vi "ZyklussteuerungGV-05-17.vi"(0 "Traps/MachKoeff0":dbl[](array[numeric]), 1 "DIOsNummern":cluster{"DIOsMod2BNr":i32[]}[](array[cluster]), 2 "error in":errorcluster, 5 "Traps/MachKoeff1":dbl[](array[numeric]), 9 "Traps/MachKoeff2":dbl[](array[numeric]), 11 "Schieberegister":T1, 12 "Zeitpunkte/Setpoints":T3 {"FPGAPID"."proportional gain (Kc)" format="%.11g"; "FPGAPID"."integral gain (Kc*Ts/Ti)" format="%.11g"; "FPGAPID"."derivative gain (Kc*Td/Ts)" format="%.11g"}, 13 "FPGA VI Reference In":refnum<k20>, 14 "MachKoeffs":T2) -> (4 "Schieberegister":T1, 8 "error out":errorcluster)   [LabVIEW 2010]
uses:
  <vilib>/rvi/errors/niLvFpgaWhatHappensToTopLevelVI.ctl
  <vilib>/rvi/interface/common/niFpgaNodeNameForErrorReporting.ctl
  <vilib>/rvi/errors/niLvFpgaAdjustHostInterfaceError.vi
  <vilib>/rvi/interface/nirviReadWriteControl/nirviReadWriteControl.xnode
  GVZwangs.vi
  GVHorstSP.vi
  GVHeizenLH.vi
  GVVentilposition.vi
  GVZeitenZyklen.vi
  GVZwangsMPV.vi
  GVZwangsMPVPos.vi
  C:/Users/HAGAR-IV/Desktop/Zeugs/Johnny/pertrasgc fpga/FPGA-Programm-05-17.vi
  <vilib>/RVI Host/nirviSupport.llb/nirviErrorClusterFromErrorCode.vi
  C:/Users/HAGAR-IV/Desktop/Zeugs/markus/version feb 2012/FPGA Bitfiles/pertrasgcfpga2_FPGATarget_FPGA-Programm-05_A75D3647.lvbitx
  NiFpgaLv.dll
  <vilib>/Utility/error.llb/Error Cluster From Error Code.vi
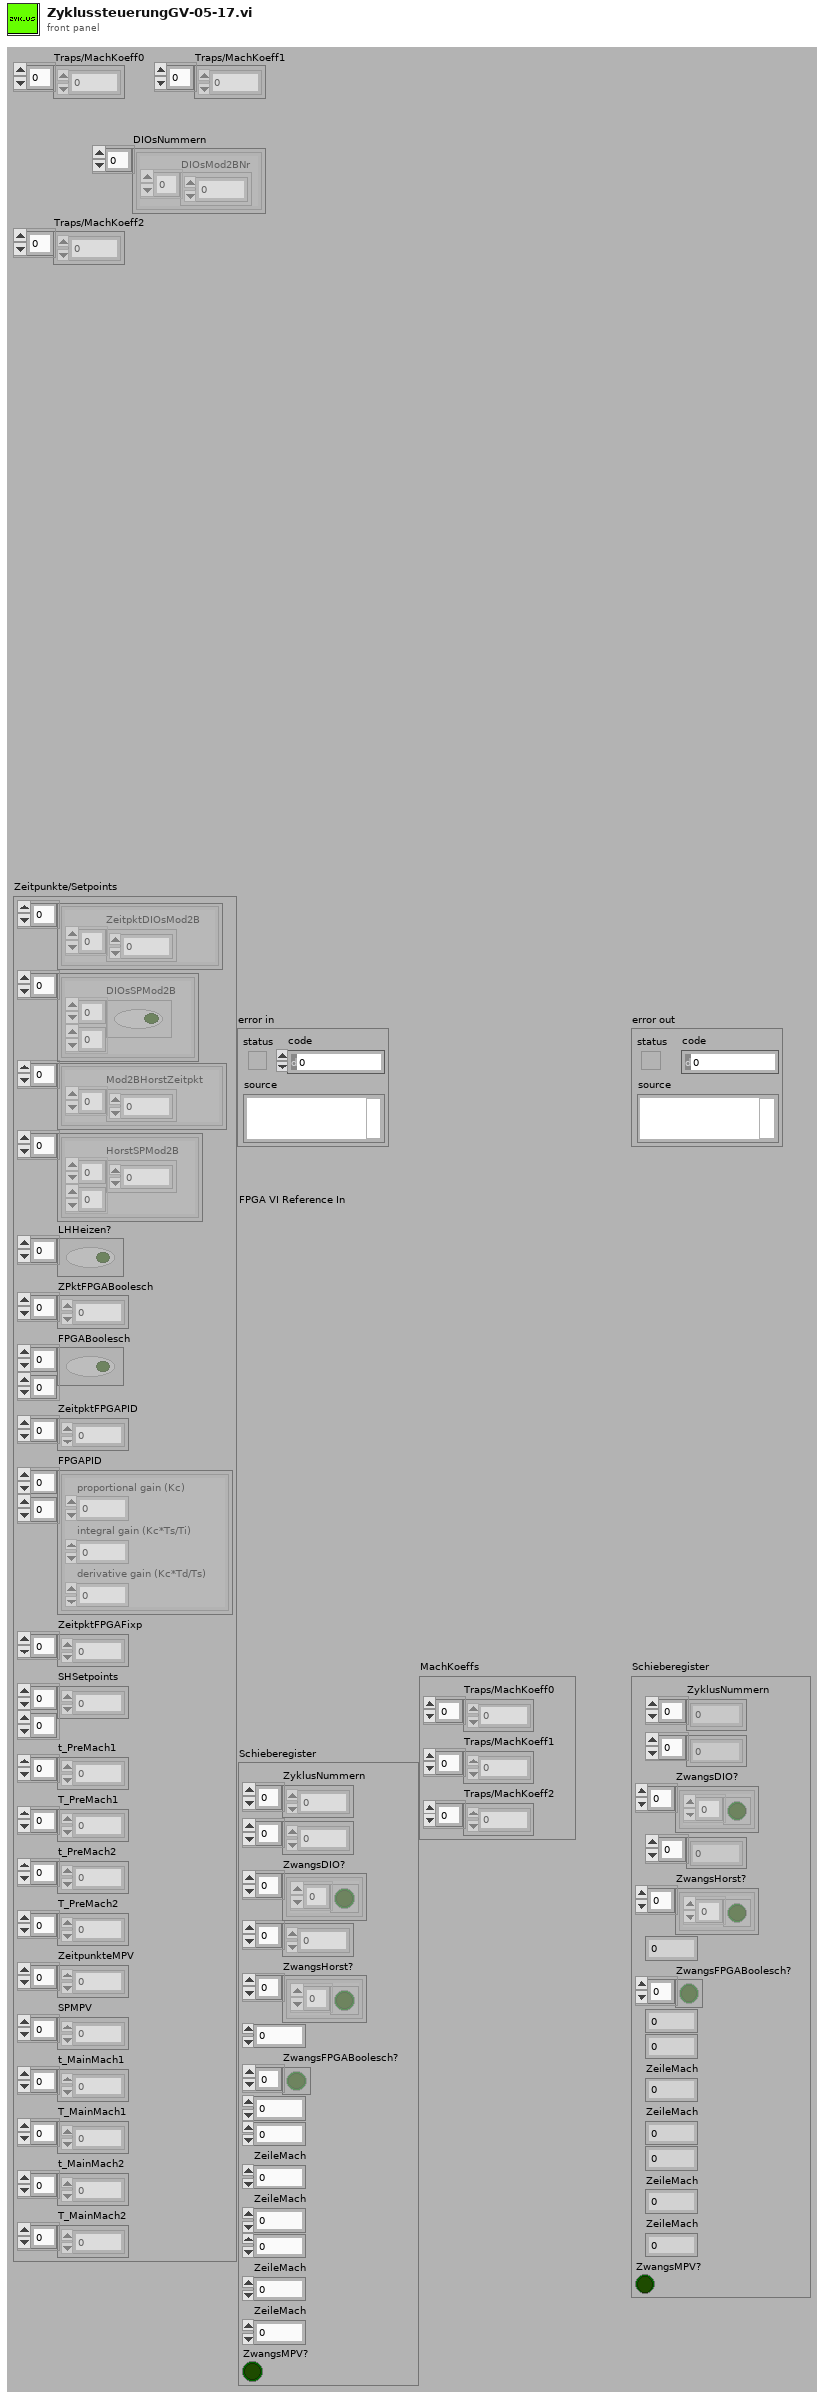
[diagram p1: front panel]
types:
  T1 = cluster{"ZyklusNummern":i32[], i32[], "ZwangsDIO?":cluster{bool[]}[], i32[], "ZwangsHorst?":cluster{bool[]}[], i32, "ZwangsFPGABoolesch?":bool[], i32, i32, "ZeileMach":i32, "ZeileMach":i32, i32, "ZeileMach":i32, "ZeileMach":i32, "ZwangsMPV?":bool}
  T2 = cluster{"Traps/MachKoeff0":dbl[], "Traps/MachKoeff1":dbl[], "Traps/MachKoeff2":dbl[]}
  T3 = cluster{cluster{"ZeitpktDIOsMod2B":dbl[]}[], cluster{"DIOsSPMod2B":bool[][]}[], cluster{"Mod2BHorstZeitpkt":dbl[]}[], cluster{"HorstSPMod2B":dbl[][]}[], "LHHeizen?":bool[], "ZPktFPGABoolesch":dbl[], "FPGABoolesch":bool[][], "ZeitpktFPGAPID":dbl[], "FPGAPID":cluster{"proportional gain (Kc)":fxp<+/-,16,8>, "integral gain (Kc*Ts/Ti)":fxp<+/-,16,8>, "derivative gain (Kc*Td/Ts)":fxp<+/-,16,8>}[][], "ZeitpktFPGAFixp":dbl[], "SHSetpoints":dbl[][], "t_PreMach1":dbl[], "T_PreMach1":dbl[], "t_PreMach2":dbl[], "T_PreMach2":dbl[], "ZeitpunkteMPV":dbl[], "SPMPV":i32[], "t_MainMach1":dbl[], "T_MainMach1":dbl[], "t_MainMach2":dbl[], "T_MainMach2":dbl[]}
  T4 = cluster{"proportional gain (Kc)":fxp<+/-,16,8>, "integral gain (Kc*Ts/Ti)":fxp<+/-,16,8>, "derivative gain (Kc*Td/Ts)":fxp<+/-,16,8>}[][]
  T5 = typedef "niFpgaNodeNameForErrorReporting.ctl" = enum16{"Open FPGA VI Reference", "Read/Write Control", "Invoke Method: Abort", "Invoke Method: Acknowledge IRQ", "Invoke Method: Download", "Invoke Method: FIFO.Configure", "Invoke Method: FIFO.Read", "Invoke Method: FIFO.Start", "Invoke Method: FIFO.Stop", "Invoke Method: FIFO.Write", "Invoke Method: Reset", "Invoke Method: Run", "Invoke Method: Wait on IRQ", "Close FPGA VI Reference"}
  T6 = typedef "niLvFpgaWhatHappensToTopLevelVI.ctl" = enum16{"top level VI scripted behind XNode", "top level VI inlined behind XNode"}
  T7 = cluster{"[0]":bool, "[1]":bool, "[2]":bool, "[3]":bool, "[4]":bool, "[5]":bool, "[6]":bool, "[7]":bool, "[8]":bool, "[9]":bool, "[10]":bool, "[11]":bool, "[12]":bool, "[13]":bool, "[14]":bool, "[15]":bool, "[16]":bool, "[17]":bool, "[18]":bool, "[19]":bool, "[20]":bool, "[21]":bool, "[22]":bool, "[23]":bool, "[24]":bool, "[25]":bool, "[26]":bool, "[27]":bool, "[28]":bool, "[29]":bool, "[30]":bool, "[31]":bool}
  T8 = cluster{"[0]":bool, "[1]":bool, "[2]":bool, "[3]":bool, "[4]":bool, "[5]":bool}
  T9 = cluster{"proportional gain (Kc)":fxp<+/-,16,8>, "integral gain (Kc*Ts/Ti)":fxp<+/-,16,8>, "derivative gain (Kc*Td/Ts)":fxp<+/-,16,8>}[]
  T10 = cluster{"FPGAPID[0]":cluster{"proportional gain (Kc)":fxp<+/-,16,8>, "integral gain (Kc*Ts/Ti)":fxp<+/-,16,8>, "derivative gain (Kc*Td/Ts)":fxp<+/-,16,8>}, "FPGAPID[1]":cluster{"proportional gain (Kc)":fxp<+/-,16,8>, "integral gain (Kc*Ts/Ti)":fxp<+/-,16,8>, "derivative gain (Kc*Td/Ts)":fxp<+/-,16,8>}, "FPGAPID[2]":cluster{"proportional gain (Kc)":fxp<+/-,16,8>, "integral gain (Kc*Ts/Ti)":fxp<+/-,16,8>, "derivative gain (Kc*Td/Ts)":fxp<+/-,16,8>}, "FPGAPID[3]":cluster{"proportional gain (Kc)":fxp<+/-,16,8>, "integral gain (Kc*Ts/Ti)":fxp<+/-,16,8>, "derivative gain (Kc*Td/Ts)":fxp<+/-,16,8>}, "FPGAPID[4]":cluster{"proportional gain (Kc)":fxp<+/-,16,8>, "integral gain (Kc*Ts/Ti)":fxp<+/-,16,8>, "derivative gain (Kc*Td/Ts)":fxp<+/-,16,8>}, "FPGAPID[5]":cluster{"proportional gain (Kc)":fxp<+/-,16,8>, "integral gain (Kc*Ts/Ti)":fxp<+/-,16,8>, "derivative gain (Kc*Td/Ts)":fxp<+/-,16,8>}}
  T11 = cluster{"proportional gain (Kc)":fxp<+/-,16,8>, "integral gain (Kc*Ts/Ti)":fxp<+/-,16,8>, "derivative gain (Kc*Td/Ts)":fxp<+/-,16,8>}
  T12 = cluster{"USetp [V]Mach1":fxp<+/-,16,6>, "[1]":fxp<+/-,16,4>, "[2]":fxp<+/-,16,4>, "[3]":fxp<+/-,16,4>, "[4]":fxp<+/-,16,4>, "[5]":fxp<+/-,16,4>, "[6]":fxp<+/-,16,4>, "[7]":fxp<+/-,16,4>, "[8]":fxp<+/-,16,4>}
  T13 = cluster{"SpannungenSH[V][0]":fxp<+/-,16,4>, "SpannungenSH[V][1]":fxp<+/-,16,4>, "SpannungenSH[V][2]":fxp<+/-,16,4>, "SpannungenSH[V][3]":fxp<+/-,16,4>}
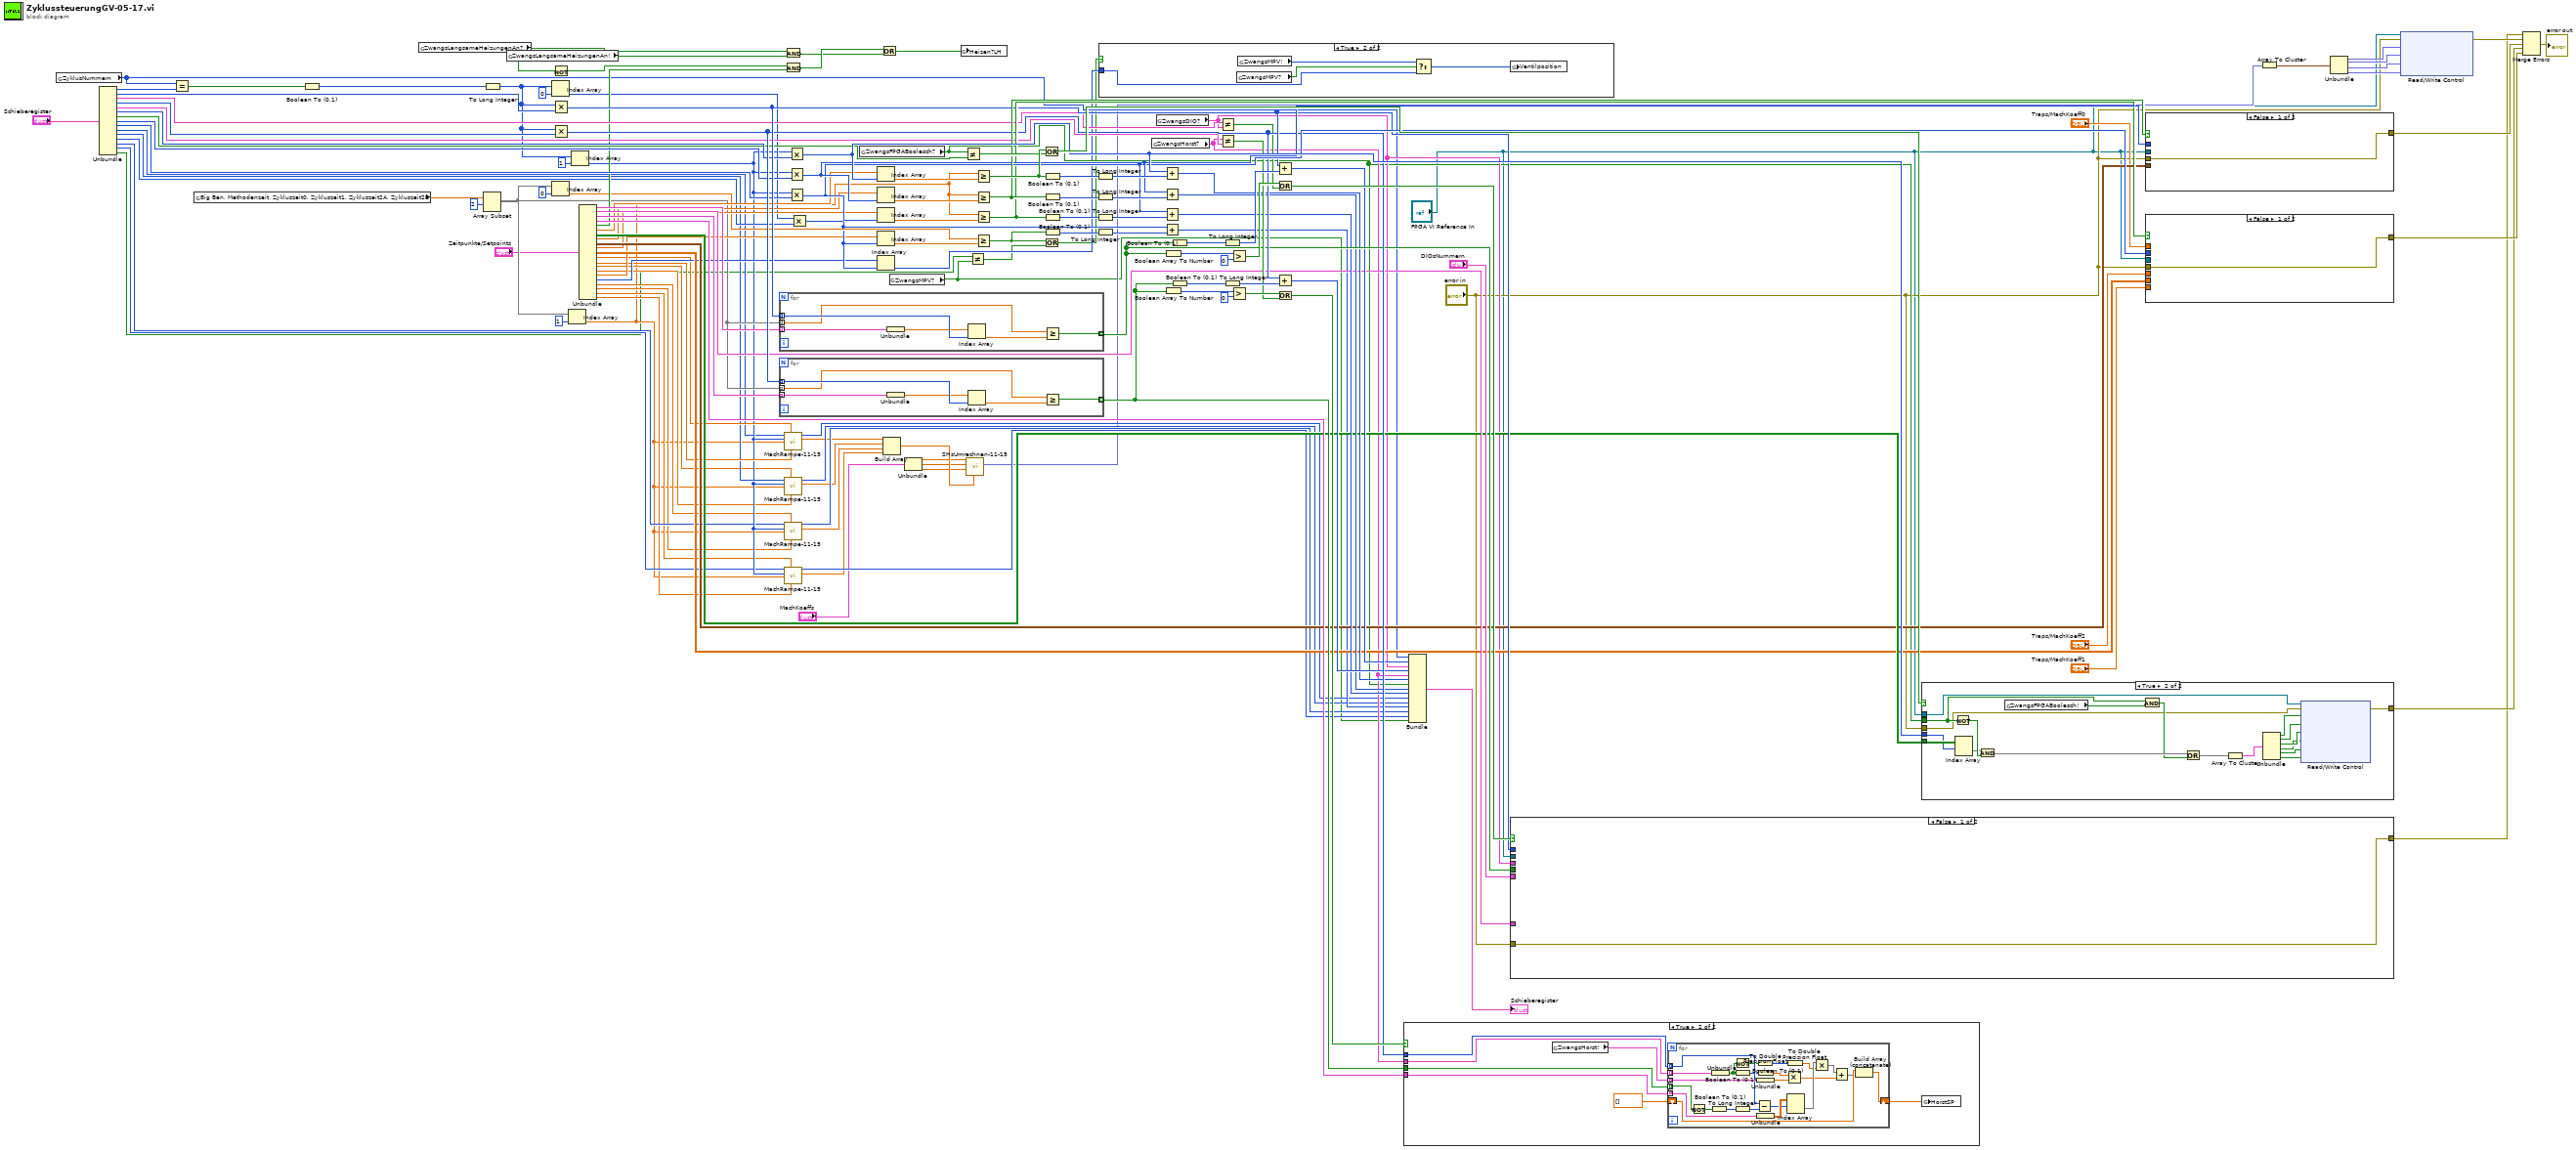
[diagram p0: block diagram]
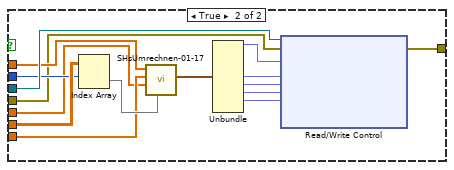
[diagram p4: hidden frame]
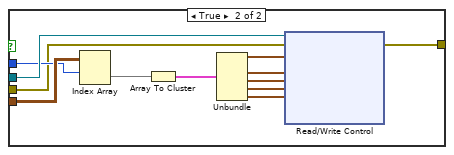
[diagram p5: hidden frame]
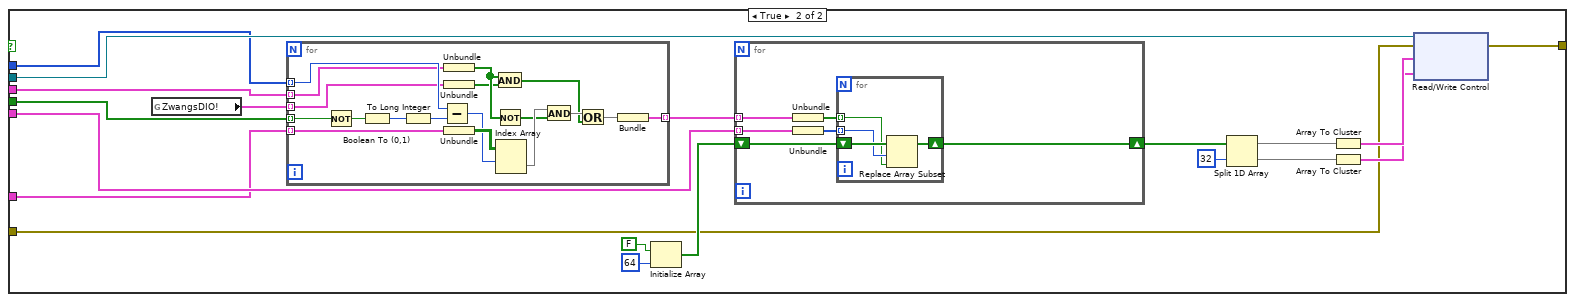
[diagram p7: hidden frame]
diagram:
  n1 = global read "GVZeitenZyklen.vi" "ZyklusNummern"() -> (w57:i32[])
  n2 = Unbundle("Schieberegister") -> ("ZyklusNummern"=w101:i32[], w100:i32[], "ZwangsDIO?"=w99:cluster{bool[]}[], w98:i32[], "ZwangsHorst?"=w97:cluster{bool[]}[], w96:i32, "ZwangsFPGABoolesch?"=w95:bool[], w94:i32, w93:i32, "ZeileMach"=w34:i32, "ZeileMach"=w49:i32, w60:i32, "ZeileMach"=w47:i32, "ZeileMach"=w46:i32, "ZwangsMPV?"=w12:bool)
  n3 = Equal?(x=w57, y=w101) -> (x = y?=w144:bool[])
  n4 = global read "GVZeitenZyklen.vi" "Big Ben, Methodenzeit, Zykluszeit0, Zykluszeit1, Zykluszeit2A, Zykluszeit2B"() -> (w55:dbl[])
  n5 = Boolean To (0,1)(Boolean=w144) -> (0, 1=w143:i16[])
  n6 = global read "GVZwangs.vi" "ZwangsLangsameHeizungenAn?"() -> (w74:bool[])
  n7 = Array Subset(array=w55, index=2 ("Index")) -> (w54:dbl[])  [unwired: 1 in]
  n8 = To Long Integer(number=w143) -> (32bit integer=w70:i32[])
  n9 = global read "GVZwangs.vi" "ZwangsLangsameHeizungenAn!"() -> (w73:bool[])
  n10 = Index Array(array=w70, index=0 ("Index")) -> (element=w68:i32)
  n11 = Index Array(array=w54, index=0 ("Index")) -> (element=w65:dbl)
  n12 = Not(x=w74) -> (.not. x?=w112:bool[])
  n13 = Multiply(x=w70, y=w100) -> (x*y=w109:i32[])
  n14 = Multiply(x=w70, y=w98) -> (x*y=w106:i32[])
  n15 = Index Array(array=w54, index=1 ("Index")) -> (element=w35:dbl)
  n16 = Index Array(array=w70, index=1 ("Index")) -> (element=w48:i32)
  n17 = Unbundle("Zeitpunkte/Setpoints") -> (w87:cluster{"ZeitpktDIOsMod2B":dbl[]}[], w86:cluster{"DIOsSPMod2B":bool[][]}[], w85:cluster{"Mod2BHorstZeitpkt":dbl[]}[], w84:cluster{"HorstSPMod2B":dbl[][]}[], "LHHeizen?"=w83:bool[], "ZPktFPGABoolesch"=w82:dbl[], "FPGABoolesch"=w81:bool[][], "ZeitpktFPGAPID"=w80:dbl[], "FPGAPID"=w79:T4, "ZeitpktFPGAFixp"=w78:dbl[], "SHSetpoints"=w77:dbl[][], "t_PreMach1"=w52:dbl[], "T_PreMach1"=w51:dbl[], "t_PreMach2"=w45:dbl[], "T_PreMach2"=w44:dbl[], "ZeitpunkteMPV"=w59:dbl[], "SPMPV"=w58:i32[], "t_MainMach1"=w43:dbl[], "T_MainMach1"=w42:dbl[], "t_MainMach2"=w41:dbl[], "T_MainMach2"=w40:dbl[])
  n18 = for {
    tunnel: w109 -> [w150] mode=indexing
    tunnel: w54 -> [w149] mode=indexing
    tunnel: [w148] -> w103 mode=indexing
    tunnel: w87 -> [w146] mode=indexing
    n19 = Unbundle(w146) -> ("ZeitpktDIOsMod2B"=w145:dbl[])
    n20 = Index Array(array=w145, index=w150) -> (element=w147:dbl)
    n21 = Greater Or Equal?(x=w149, y=w147) -> (x >= y?=w148:bool)
  }
  n22 = for {
    tunnel: w106 -> [w156] mode=indexing
    tunnel: w54 -> [w155] mode=indexing
    tunnel: w85 -> [w152] mode=indexing
    tunnel: [w153] -> w107 mode=indexing
    n23 = Unbundle(w152) -> ("Mod2BHorstZeitpkt"=w151:dbl[])
    n24 = Index Array(array=w151, index=w156) -> (element=w154:dbl)
    n25 = Greater Or Equal?(x=w155, y=w154) -> (x >= y?=w153:bool)
  }
  n26 = call "MachRampe-11-15.vi"("T_Mach"=w51, "t_Mach"=w52, "ZykluszeitMod1"=w35, "gleicherZyklus?"=w48, "ZeileMach"=w34) -> ("T_Mach"=w33:dbl, "ZeileMach"=w50:i32)  [unwired: 5 in]
  n27 = call "MachRampe-11-15.vi"("T_Mach"=w44, "t_Mach"=w45, "ZykluszeitMod1"=w35, "gleicherZyklus?"=w48, "ZeileMach"=w49) -> ("T_Mach"=w32:dbl, "ZeileMach"=w39:i32)  [unwired: 5 in]
  n28 = call "MachRampe-11-15.vi"("T_Mach"=w42, "t_Mach"=w43, "ZykluszeitMod1"=w35, "gleicherZyklus?"=w48, "ZeileMach"=w47) -> ("T_Mach"=w31:dbl, "ZeileMach"=w38:i32)  [unwired: 5 in]
  n29 = call "MachRampe-11-15.vi"("T_Mach"=w40, "t_Mach"=w41, "ZykluszeitMod1"=w35, "gleicherZyklus?"=w48, "ZeileMach"=w46) -> ("T_Mach"=w30:dbl, "ZeileMach"=w37:i32)  [unwired: 5 in]
  n30 = And(x=w74, y=w73) -> (x .and. y?=w110:bool[])
  n31 = And(x=w112, y=w83) -> (x .and. y?=w111:bool[])
  n32 = Multiply(x=w48, y=w96) -> (x*y=w123:i32)
  n33 = Multiply(x=w48, y=w94) -> (x*y=w118:i32)
  n34 = Multiply(x=w48, y=w93) -> (x*y=w114:i32)
  n35 = Multiply(x=w68, y=w60) -> (x*y=w62:i32)
  n36 = global read "GVZwangs.vi" "ZwangsFPGABoolesch?"() -> (w71:bool[])
  n37 = Index Array(array=w82, index=w123) -> (element=w129:dbl)
  n38 = Index Array(array=w80, index=w118) -> (element=w122:dbl)
  n39 = Index Array(array=w78, index=w114) -> (element=w117:dbl)
  n40 = Index Array(array=w59, index=w62) -> (element=w66:dbl)
  n41 = Index Array(array=w58, index=w62) -> (element=w15:i32)
  n42 = Or(x=w111, y=w110) -> (x .or. y?=w72:bool[])
  n43 = Build Array(w33, w32, w31, w30) -> (w29:dbl[])
  n44 = global read "GVZwangsMPV.vi" "ZwangsMPV?"() -> (w13:bool)
  n45 = Unbundle("MachKoeffs") -> ("Traps/MachKoeff0"=w24:dbl[], "Traps/MachKoeff1"=w23:dbl[], "Traps/MachKoeff2"=w22:dbl[])
  n46 = global write "GVHeizenLH.vi" "Heizen?LH"(w72) -> ()
  n47 = Not Equal?(x=w71, y=w95) -> (x != y?=w125:bool)
  n48 = call "SHsUmrechnen-11-15.vi"("TemperaturenSH[V]"=w29, "Traps/MachKoeff2"=w22, "Traps/MachKoeff1"=w23, "Traps/MachKoeff0"=w24) -> ("SpannungenSH[V]"=w21:fxp<+/-,16,4>[])  [unwired: 6 in, 1 out]
  n49 = Not Equal?(x=w12, y=w13) -> (x != y?=w11:bool)
  n50 = Greater Or Equal?(x=w35, y=w129) -> (x >= y?=w126:bool)
  n51 = Greater Or Equal?(x=w35, y=w122) -> (x >= y?=w119:bool)
  n52 = Greater Or Equal?(x=w35, y=w117) -> (x >= y?=w113:bool)
  n53 = Greater Or Equal?(x=w65, y=w66) -> (x >= y?=w10:bool)
  n54 = Or(x=w126, y=w125) -> (x .or. y?=w124:bool)
  n55 = Or(x=w10, y=w11) -> (x .or. y?=w9:bool)
  n56 = Boolean To (0,1)(Boolean=w126) -> (0, 1=w128:i16)
  n57 = Boolean To (0,1)(Boolean=w119) -> (0, 1=w121:i16)
  n58 = Boolean To (0,1)(Boolean=w113) -> (0, 1=w116:i16)
  n59 = Boolean To (0,1)(Boolean=w10) -> (0, 1=w64:i16)
  n60 = To Long Integer(number=w128) -> (32bit integer=w127:i32)
  n61 = To Long Integer(number=w121) -> (32bit integer=w120:i32)
  n62 = To Long Integer(number=w116) -> (32bit integer=w115:i32)
  n63 = To Long Integer(number=w64) -> (32bit integer=w63:i32)
  n64 = case shown="True" w9 {
    tunnel: w15 -> [_ w158]
    frame False {
    }
    frame True {
      n65 = global read "GVZwangsMPV.vi" "ZwangsMPV?"() -> (w160:bool)
      n66 = global read "GVZwangsMPVPos.vi" "ZwangsMPV!"() -> (w159:i32)
      n67 = Select(t=w159, s=w160, f=w158) -> (s? t:f=w157:i32)
      n68 = global write "GVVentilposition.vi" "Ventilposition"(w157) -> ()
    }
  }
  n69 = global read "GVZwangs.vi" "ZwangsHorst?"() -> (w75:cluster{bool[]}[])
  n70 = global read "GVZwangs.vi" "ZwangsDIO?"() -> (w76:cluster{bool[]}[])
  n71 = Add(x=w123, y=w127) -> (x+y=w90:i32)
  n72 = Add(x=w118, y=w120) -> (x+y=w89:i32)
  n73 = Add(x=w114, y=w115) -> (x+y=w88:i32)
  n74 = Add(x=w62, y=w63) -> (x+y=w61:i32)
  n75 = Boolean Array To Number(Boolean array=w103) -> (number=w140:u32)
  n76 = Boolean Array To Number(Boolean array=w107) -> (number=w134:u32)
  n77 = Boolean To (0,1)(Boolean=w103) -> (0, 1=w142:i16[])
  n78 = Boolean To (0,1)(Boolean=w107) -> (0, 1=w136:i16[])
  n79 = Not Equal?(x=w99, y=w76) -> (x != y?=w104:bool)
  n80 = Not Equal?(x=w75, y=w97) -> (x != y?=w105:bool)
  n81 = To Long Integer(number=w142) -> (32bit integer=w141:i32[])
  n82 = To Long Integer(number=w136) -> (32bit integer=w135:i32[])
  n83 = Greater?(x=w140, y=u32 0) -> (0:w137:bool)
  n84 = Greater?(x=w134, y=u32 0) -> (0:w132:bool)
  n85 = Add(x=w109, y=w141) -> (x+y=w92:i32[])
  n86 = Or(x=w137, y=w104) -> (x .or. y?=w138:bool)
  n87 = Add(x=w106, y=w135) -> (x+y=w91:i32[])
  n88 = Or(x=w132, y=w105) -> (x .or. y?=w108:bool)
  n89 = case shown="True" w108 {
    tunnel: w84 -> [_ w164]
    tunnel: w75 -> [_ w165]
    tunnel: w107 -> [_ w167]
    tunnel: w106 -> [_ w166]
    frame False {
    }
    frame True {
      n90 = global read "GVZwangs.vi" "ZwangsHorst!"() -> (w162:cluster{dbl[]}[])
      n91 = for {
        tunnel: w167 -> [w187] mode=indexing
        tunnel: w166 -> [w184] mode=indexing
        tunnel: w165 -> [w190] mode=indexing
        tunnel: w164 -> [w188] mode=indexing
        tunnel: w162 -> [w189] mode=indexing
        shift-right: [w168] -> w161
        shift-left: dbl[] [] -> [w170]
        n92 = Not(x=w187) -> (.not. x?=w186:bool)
        n93 = Boolean To (0,1)(Boolean=w186) -> (0, 1=w185:i16)
        n94 = Unbundle(w190) -> (w177:bool[])
        n95 = Not(x=w177) -> (.not. x?=w180:bool[])
        n96 = Boolean To (0,1)(Boolean=w177) -> (0, 1=w178:i16[])
        n97 = To Long Integer(number=w185) -> (32bit integer=w183:i32)
        n98 = Subtract(x=w184, y=w183) -> (x-y=w181:i32)
        n99 = Boolean To (0,1)(Boolean=w180) -> (0, 1=w179:i16[])
        n100 = To Double Precision Float(number=w178) -> (double precision float=w174:dbl[])
        n101 = Unbundle(w189) -> (w173:dbl[])
        n102 = Unbundle(w188) -> ("HorstSPMod2B"=w182:dbl[][])
        n103 = Multiply(x=w174, y=w173) -> (x*y=w171:dbl[])
        n104 = To Double Precision Float(number=w179) -> (double precision float=w175:dbl[])
        n105 = Index Array(array=w182, index (row)=w181) -> (element=w176:dbl[])  [unwired: 1 in]
        n106 = Multiply(x=w176, y=w175) -> (x*y=w172:dbl[])
        n107 = Add(x=w172, y=w171) -> (x+y=w169:dbl[])
        n108 = Build Array (concatenate)(w170, w169) -> (w168:dbl[])
      }
      n109 = global write "GVHorstSP.vi" "HorstSP"(w161) -> ()
    }
  }
  n110 = Bundle("ZyklusNummern"=w57, w92, "ZwangsDIO?"=w76, w91, "ZwangsHorst?"=w75, w90, "ZwangsFPGABoolesch?"=w71, w89, w88, "ZeileMach"=w50, "ZeileMach"=w39, w61, "ZeileMach"=w38, "ZeileMach"=w37, "ZwangsMPV?"=w13) -> (→"Schieberegister":T1)  [unwired: 1 in]
  n111 = case shown="False" w138 {
    tunnel: w109 -> [_ w206]
    tunnel: w76 -> [_ w203]
    tunnel: "DIOsNummern" -> [_ w210]
    tunnel: "FPGA VI Reference In" -> [_ w209]
    tunnel: w86 -> [_ w204]
    tunnel: w103 -> [_ w205]
    tunnel: "error in" -> [w191 w193]
    tunnel: [w191 w192] -> w3
    frame False {
    }
    frame True {
      n112 = global read "GVZwangs.vi" "ZwangsDIO!"() -> (w194:cluster{bool[]}[])
      n113 = for {
        tunnel: w206 -> [w225] mode=indexing
        tunnel: w205 -> [w224] mode=indexing
        tunnel: w204 -> [w223] mode=indexing
        tunnel: w203 -> [w222] mode=indexing
        tunnel: w194 -> [w221] mode=indexing
        tunnel: [w211] -> w202 mode=indexing
        n114 = Not(x=w224) -> (.not. x?=w227:bool)
        n115 = Boolean To (0,1)(Boolean=w227) -> (0, 1=w226:i16)
        n116 = To Long Integer(number=w226) -> (32bit integer=w228:i32)
        n117 = Subtract(x=w225, y=w228) -> (x-y=w219:i32)
        n118 = Unbundle(w222) -> (w216:bool[])
        n119 = Unbundle(w221) -> (w215:bool[])
        n120 = Unbundle(w223) -> ("DIOsSPMod2B"=w220:bool[][])
        n121 = And(x=w216, y=w215) -> (x .and. y?=w213:bool[])
        n122 = Not(x=w216) -> (.not. x?=w217:bool[])
        n123 = Index Array(array=w220, index (row)=w219) -> (element=w218:bool[])  [unwired: 1 in]
        n124 = And(x=w218, y=w217) -> (x .and. y?=w214:bool[])
        n125 = Or(x=w214, y=w213) -> (x .or. y?=w212:bool[])
        n126 = Bundle(w212) -> (w211:cluster{bool[]})  [unwired: 1 in]
      }
      n127 = Initialize Array(FALSE, 64 ("Dimension")) -> (w195:bool[])
      n128 = for {
        tunnel: w202 -> [w256] mode=indexing
        tunnel: w210 -> [w258] mode=indexing
        shift-right: [w259] -> w207
        shift-left: w195 -> [w260]
        n129 = Unbundle(w256) -> (w255:bool[])
        n130 = Unbundle(w258) -> ("DIOsMod2BNr"=w257:i32[])
        n131 = for {
          tunnel: w255 -> [w262] mode=indexing
          tunnel: w257 -> [w263] mode=indexing
          shift-right: [w261] -> w259
          shift-left: w260 -> [w264]
          n132 = Replace Array Subset(array=w264, new element=w262, index=w263) -> (w261:bool[])
        }
      }
      n133 = Split 1D Array(array=w207, index=32 ("Länge")) -> (first subarray=w201:bool[], second subarray=w199:bool[])
      n134 = Array To Cluster(array=w201) -> (cluster=w200:T7)
      n135 = Array To Cluster(array=w199) -> (cluster=w198:T7)
      n136 = xnode "Read/Write Control"("FPGA VI Reference In"=w209, "error in"=w193, "Mod5/DIO"=w200, "Mod6/DIO"=w198) -> ("error out"=w192:errorcluster)  [unwired: 1 out]
    }
  }
  n137 = case shown="True" w124 {
    tunnel: w123 -> [_ w275]
    tunnel: w71 -> [_ w280]
    tunnel: w81 -> [_ w284]
    tunnel: "FPGA VI Reference In" -> [_ w277]
    tunnel: "error in" -> [w265 w273]
    tunnel: [w265 w272] -> w7
    frame False {
    }
    frame True {
      n138 = Not(x=w280) -> (.not. x?=w283:bool[])
      n139 = Index Array(array=w284, index (row)=w275) -> (element=w282:bool[])  [unwired: 1 in]
      n140 = And(x=w282, y=w283) -> (x .and. y?=w281:bool[])
      n141 = global read "GVZwangs.vi" "ZwangsFPGABoolesch!"() -> (w274:bool[])
      n142 = And(x=w280, y=w274) -> (x .and. y?=w279:bool[])
      n143 = Or(x=w281, y=w279) -> (x .or. y?=w278:bool[])
      n144 = Array To Cluster(array=w278) -> (cluster=w276:T8)
      n145 = Unbundle(w276) -> ("[0]"=w271:bool, "[1]"=w270:bool, "[2]"=w269:bool, "[3]"=w268:bool, "[4]"=w267:bool, "[5]"=w266:bool)
      n146 = xnode "Read/Write Control"("FPGA VI Reference In"=w277, "error in"=w273, "Heizen?Trap1"=w271, "Heizen?Trap2"=w270, "Heizen?PreMach1"=w269, "Heizen?PreMach2"=w268, "Heizen?MainMach1"=w267, "Heizen?MainMach2"=w266) -> ("error out"=w272:errorcluster)  [unwired: 1 out]
    }
  }
  n147 = case shown="False" w119 {
    tunnel: "FPGA VI Reference In" -> [_ w440]
    tunnel: w79 -> [_ w439]
    tunnel: w118 -> [_ w433]
    tunnel: "error in" -> [w428 w430]
    tunnel: [w428 w429] -> w6
    frame False {
    }
    frame True {
      n148 = Index Array(array=w439, index (row)=w433) -> (element=w438:T9)  [unwired: 1 in]
      n149 = Array To Cluster(array=w438) -> (cluster=w437:T10)
      n150 = Unbundle(w437) -> ("FPGAPID[0]"=w436:T11, "FPGAPID[2]"=w435:T11, "FPGAPID[3]"=w434:T11, "FPGAPID[4]"=w432:T11, "FPGAPID[5]"=w431:T11)  [unwired: 1 out]
      n151 = xnode "Read/Write Control"("FPGA VI Reference In"=w440, "error in"=w430, "PIDTrap1"=w436, "PIDPreMach1"=w435, "PIDPreMach2"=w434, "PIDMainMach1"=w432, "PIDMainMach2"=w431) -> ("error out"=w429:errorcluster)  [unwired: 1 out]
    }
  }
  n152 = case shown="False" w113 {
    tunnel: w114 -> [_ w495]
    tunnel: w77 -> [_ w497]
    tunnel: "FPGA VI Reference In" -> [_ w496]
    tunnel: "Traps/MachKoeff2" -> [_ w485]
    tunnel: "Traps/MachKoeff1" -> [_ w486]
    tunnel: "Traps/MachKoeff0" -> [_ w487]
    tunnel: "error in" -> [w482 w484]
    tunnel: [w482 w483] -> w8
    frame False {
    }
    frame True {
      n153 = Index Array(array=w497, index (row)=w495) -> (element=w488:dbl[])  [unwired: 1 in]
      n154 = call "SHsUmrechnen-01-17.vi"("TemperaturenSH[V]"=w488, "Traps/MachKoeff2"=w485, "Traps/MachKoeff1"=w486, "Traps/MachKoeff0"=w487) -> ("Spannungen SH"=w489:T12)  [unwired: 6 in, 1 out]
      n155 = Unbundle(w489) -> ("USetp [V]Mach1"=w494:fxp<+/-,16,6>, "[4]"=w493:fxp<+/-,16,4>, "[5]"=w492:fxp<+/-,16,4>, "[6]"=w491:fxp<+/-,16,4>, "[7]"=w490:fxp<+/-,16,4>)  [unwired: 4 out]
      n156 = xnode "Read/Write Control"("FPGA VI Reference In"=w496, "error in"=w484, "SetpointTrap1"=w494, "Umax[V]PreMach1"=w493, "Umax[V]PreMach2"=w492, "Umax[V]MainMach1"=w491, "Umax[V]MainMach2"=w490) -> ("error out"=w483:errorcluster)  [unwired: 1 out]
    }
  }
  n157 = Array To Cluster(array=w21) -> (cluster=w20:T13)
  n158 = Unbundle(w20) -> ("SpannungenSH[V][0]"=w19:fxp<+/-,16,4>, "SpannungenSH[V][1]"=w18:fxp<+/-,16,4>, "SpannungenSH[V][2]"=w17:fxp<+/-,16,4>, "SpannungenSH[V][3]"=w16:fxp<+/-,16,4>)
  n159 = xnode "Read/Write Control"("FPGA VI Reference In"="FPGA VI Reference In", "error in"="error in", "USetp[V]PreMach1"=w19, "USetp[V]PreMach2"=w18, "USetp[V]MainMach1"=w17, "USetp[V]MainMach2"=w16) -> ("error out"=w5:errorcluster)  [unwired: 1 out]
  n160 = Merge Errors(w3, w5, w6, w7, w8) -> (→"error out":errorcluster)
